vi "ctet_dmm_User Main.vi"() -> ()   [LabVIEW 2019, in "ctet_dmm User Library.lvlib"]
uses:
  ctet_dmm User Library.lvlib
  Servers/ctet_dmm/ctet_dmm Class/typeDefs/Server State Data.ctl
  Servers/ctet_dmm/ctet_dmm Class/ctet_dmm.lvclass/ctet_dmm.ctl
  Servers/ctet_dmm/ctet_dmm Class/ctet_dmm.lvclass
panel:
  in  "Stop":bool
  in  "Server Address":string="0.0.0.0:50051"
  in  "Server Certificate File (.crt)":path
  in  "Server Key File (.key)":path
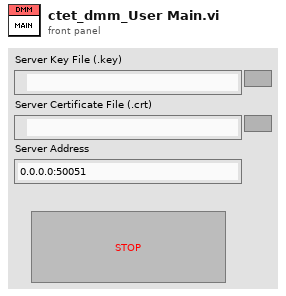
[diagram p1: front panel]
types:
  T1 = typedef "ctet_dmm.lvlib/ctet_dmm.lvclass/Server State Data.ctl" = cluster{"Data":string}
  T2 = typedef "ctet_dmm.lvlib/ctet_dmm.lvclass/Server gRPC UEs.ctl" = cluster{"Invoke gRPC UE":refnum<user-event>, "Query gRPC UE":refnum<user-event>, "Register gRPC UE":refnum<user-event>, "OpenDMMSession gRPC UE":refnum<user-event>, "ConfigureDMM gRPC UE":refnum<user-event>, "PerformDMMVoltageMeasurement gRPC UE":refnum<user-event>, "CloseDMMSession gRPC UE":refnum<user-event>, "SelfCalibrateDMM gRPC UE":refnum<user-event>, "ResetDMM gRPC UE":refnum<user-event>}
  T3 = typedef "ctet_dmm.lvlib/gprc-lvsupport.lvlib/grpcId.ctl" = u64
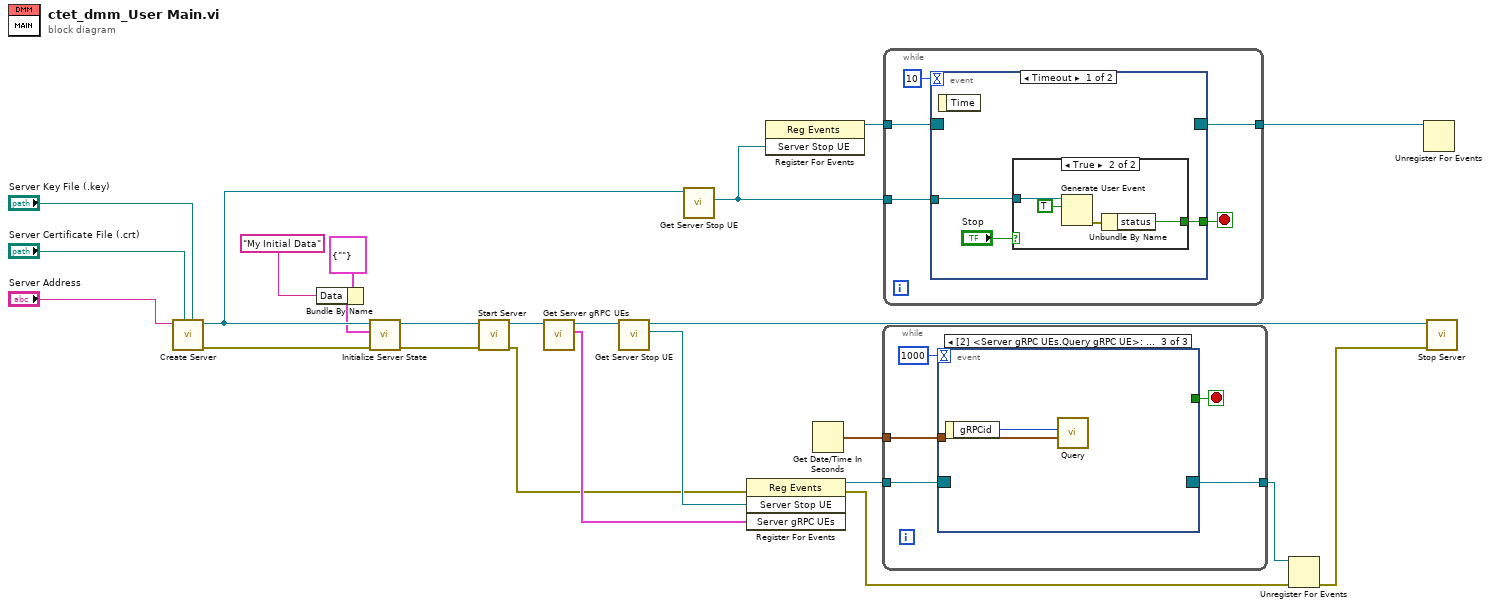
[diagram p0: block diagram]
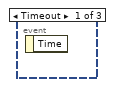
[diagram p2: hidden frame]
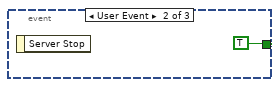
[diagram p3: hidden frame]
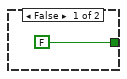
[diagram p4: hidden frame]
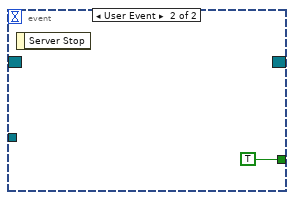
[diagram p5: hidden frame]
diagram:
  n1 = call "Create Server.vi"("Server Key File (.key)"="Server Key File (.key)", "Server Certificate File (.crt)"="Server Certificate File (.crt)", "Server Address"="Server Address") -> ("error out"=w18:errorcluster, "gRPC Server out"=w15:refnum<class "ctet_dmm.lvclass">)  [unwired: 7 in]
  n2 = Bundle By Name(cluster=T1 {"Data"=""} ("Initial State"), "Data"="My Initial Data") -> (w13:T1)
  n3 = call "Initialize Server State.vi"("error in (no error)"=w18, "Initial State"=w13, "gRPC Server in"=w15) -> ("error out"=w17:errorcluster, "gRPC Server out"=w16:refnum<class "ctet_dmm.lvclass">)  [unwired: 7 in]
  n4 = call "Start Server.vi"("error in (no error)"=w17, "gRPC Server in"=w16) -> ("error out"=w5:errorcluster, "gRPC Server out"=w6:refnum<class "ctet_dmm.lvclass">)  [unwired: 8 in]
  n5 = call "Get Server gRPC UEs.vi"("OOP Server in"=w6) -> ("Server gRPC UEs"=w9:T2, "OOP Server out"=w11:refnum<class "ctet_dmm.lvclass">)  [unwired: 9 in]
  n6 = call "Get Server Stop UE.vi"("OOP Server in"=w11) -> ("Server Stop UE"=w10:refnum<user-event>, "OOP Server out"=w2:refnum<class "ctet_dmm.lvclass">)  [unwired: 9 in]
  n7 = call "Get Server Stop UE.vi"("OOP Server in"=w15) -> ("Server Stop UE"=w19:refnum<user-event>)  [unwired: 9 in, 1 out]
  n8 = register-events(error in=w5, w10, w9) -> (reference out=w8:refnum<event-registration>, error out=w4:errorcluster)  [unwired: 1 in]
  n9 = register-events(w19) -> (reference out=w21:refnum<event-registration>)  [unwired: 2 in, 1 out]
  n10 = Get Date/Time In Seconds() -> (seconds since 1Jan1904=w1:timestamp)
  n11 = while {
    tunnel: w8 -> [w29]
    tunnel: [w27] -> w7
    tunnel: w1 -> [w25]
    stop <- w28 stop-if-true
    n12 = event "RPC Methods Event Structure" shown="[2] <Server gRPC UEs.Query gRPC UE>: User Event" {
      selector: w29 -> [_ _ _]
      dyn-events: [_ _ _] -> w27
      timeout: 1000 -> [_ _ _]
      tunnel: [_ TRUE _] -> w28
      tunnel: w25 -> [_ _ w31]
      event Timeout {
        n13 = event-data() -> ()  [unwired: 1 in, 1 out]
      }
      event User Event {
        n14 = event-data() -> ()  [unwired: 1 in, 1 out]
      }
      event User Event {
        n15 = event-data() -> ("gRPCid"=w32:T3)  [unwired: 1 in]
        n16 = call "Query.vi"("current time"=w31, "gRPCid"=w32) -> ()  [unwired: 9 in, 1 out]
      }
    }
  }
  n17 = while {
    tunnel: w19 -> [w37]
    tunnel: w21 -> [w36]
    tunnel: [w34] -> w20
    stop <- w35 stop-if-true
    n18 = event shown="[0] Timeout" {
      selector: w36 -> [_ _]
      dyn-events: [_ _] -> w34
      timeout: 10 -> [_ _]
      tunnel: w37 -> [w40 _]
      tunnel: [w39 TRUE] -> w35
      event Timeout {
        n19 = event-data() -> ()  [unwired: 1 in, 1 out]
        n20 = case shown="True" "Stop" {
          tunnel: w40 -> [_ w43]
          tunnel: [FALSE ("status") w42] -> w39
          frame False {
          }
          frame True {
            n21 = Generate User Event(user event=w43, event data cluster=TRUE ("event data")) -> (error out=w44:errorcluster)  [unwired: 2 in, 1 out]
            n22 = Unbundle By Name(w44) -> ("status"=w42:bool)
          }
        }
      }
      event User Event {
        n23 = event-data() -> ()  [unwired: 1 in, 1 out]
      }
    }
  }
  n24 = Unregister For Events(event registration refnum=w7, error in=w4) -> (error out=w3:errorcluster)
  n25 = Unregister For Events(event registration refnum=w20) -> ()  [unwired: 1 in, 1 out]
  n26 = call "Stop Server.vi"("error in (no error)"=w3, "gRPC Server in"=w2) -> ()  [unwired: 9 in, 1 out]
